vi "analiza_trama.vi"(4 "Entrada":string) -> (20 "angulo servo direccion":dbl, 21 "distancia lidar frontal":dbl, 22 "distancia lidar lateral":dbl, 23 "PWM motor":dbl, 24 "bool sentido":dbl, 25 "tension bateria":dbl, 26 "corriente bateria":dbl, 27 "resto":string)   [LabVIEW 2025]
panel:
  out "trama":string
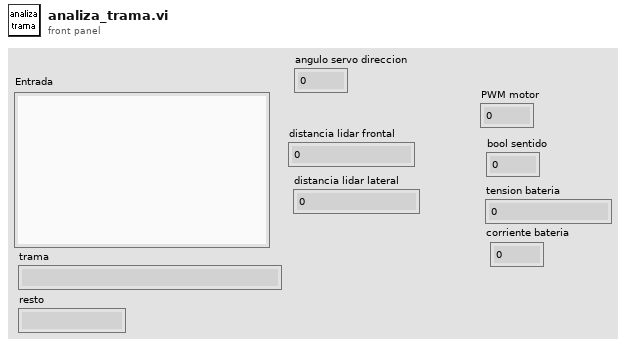
[diagram p1: front panel]
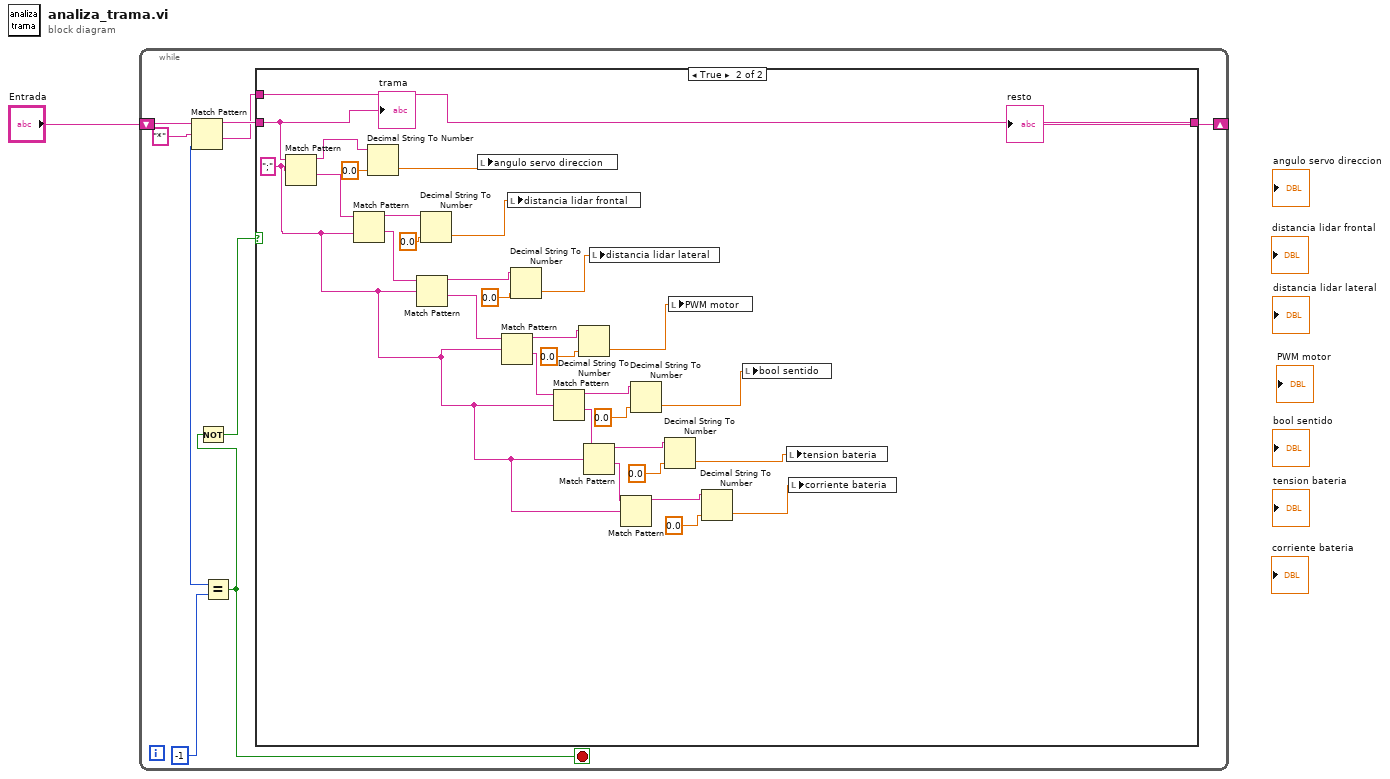
[diagram p0: block diagram]
diagram:
  n1 = while {
    shift-right: [w4] -> w1
    shift-left: "Entrada" -> [w11]
    stop <- w7 stop-if-true
    n2 = Match Pattern(string=w11, regular expression="*") -> (before substring=w5:string, after substring=w3:string, offset past match=w9:i32)  [unwired: 1 in, 1 out]
    n3 = Equal?(x=w9, y=-1) -> (x = y?=w7:bool)
    n4 = Not(x=w7) -> (.not. x?=w6:bool)
    n5 = case shown="True" w6 {
      tunnel: w5 -> [w12 w41]
      tunnel: [w12 w42] -> w4
      tunnel: w3 -> [_ w42]
      frame False {
      }
      frame True {
        w16 = ";"
        n6 = Match Pattern(string=w41, regular expression=w16) -> (before substring=w40:string, after substring=w14:string)  [unwired: 1 in, 2 out]
        n7 = Match Pattern(string=w14, regular expression=w16) -> (before substring=w38:string, after substring=w36:string)  [unwired: 1 in, 2 out]
        n8 = Decimal String To Number(string=w40, default (0L)=0.0 ("default (0 I32)")) -> (number=w21:dbl)  [unwired: 1 in, 1 out]
        n9 = Match Pattern(string=w36, regular expression=w16) -> (before substring=w35:string, after substring=w15:string)  [unwired: 1 in, 2 out]
        n10 = Decimal String To Number(string=w38, default (0L)=0.0 ("default (0 I32)")) -> (number=w13:dbl)  [unwired: 1 in, 1 out]
        n11 = local write "angulo servo direccion"(w21) -> ()
        n12 = Match Pattern(string=w15, regular expression=w16) -> (before substring=w33:string, after substring=w30:string)  [unwired: 1 in, 2 out]
        n13 = local write "distancia lidar frontal"(w13) -> ()
        n14 = Decimal String To Number(string=w35, default (0L)=0.0 ("default (0 I32)")) -> (number=w20:dbl)  [unwired: 1 in, 1 out]
        n15 = Match Pattern(string=w30, regular expression=w16) -> (before substring=w31:string, after substring=w27:string)  [unwired: 1 in, 2 out]
        n16 = Decimal String To Number(string=w33, default (0L)=0.0 ("default (0 I32)")) -> (number=w19:dbl)  [unwired: 1 in, 1 out]
        n17 = Match Pattern(string=w27, regular expression=w16) -> (before substring=w28:string, after substring=w24:string)  [unwired: 1 in, 2 out]
        n18 = local write "distancia lidar lateral"(w20) -> ()
        n19 = Match Pattern(string=w24, regular expression=w16) -> (before substring=w25:string)  [unwired: 1 in, 3 out]
        n20 = Decimal String To Number(string=w31, default (0L)=0.0 ("default (0 I32)")) -> (number=w18:dbl)  [unwired: 1 in, 1 out]
        n21 = Decimal String To Number(string=w28, default (0L)=0.0 ("default (0 I32)")) -> (number=w23:dbl)  [unwired: 1 in, 1 out]
        n22 = local write "PWM motor"(w19) -> ()
        n23 = Decimal String To Number(string=w25, default (0L)=0.0 ("default (0 I32)")) -> (number=w22:dbl)  [unwired: 1 in, 1 out]
        n24 = local write "bool sentido"(w18) -> ()
        n25 = local write "tension bateria"(w23) -> ()
        n26 = local write "corriente bateria"(w22) -> ()
        "trama" <- w41
      }
    }
  }
  "resto" <- w1
